vi "setup_lc_db.vi"(4 "shuoming":string, 6 "jsren":string, 7 "zc_luodi_num":string, 8 "didian":string, 9 "yw":string, 11 "id":string) -> (2 "error":errorcluster caption="error out 2")   [LabVIEW 2017, in "Lib_code.lvlib"]
uses:
  Lib_code.lvlib
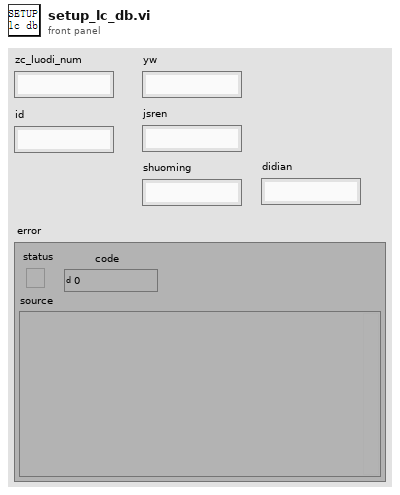
[diagram p1: front panel]
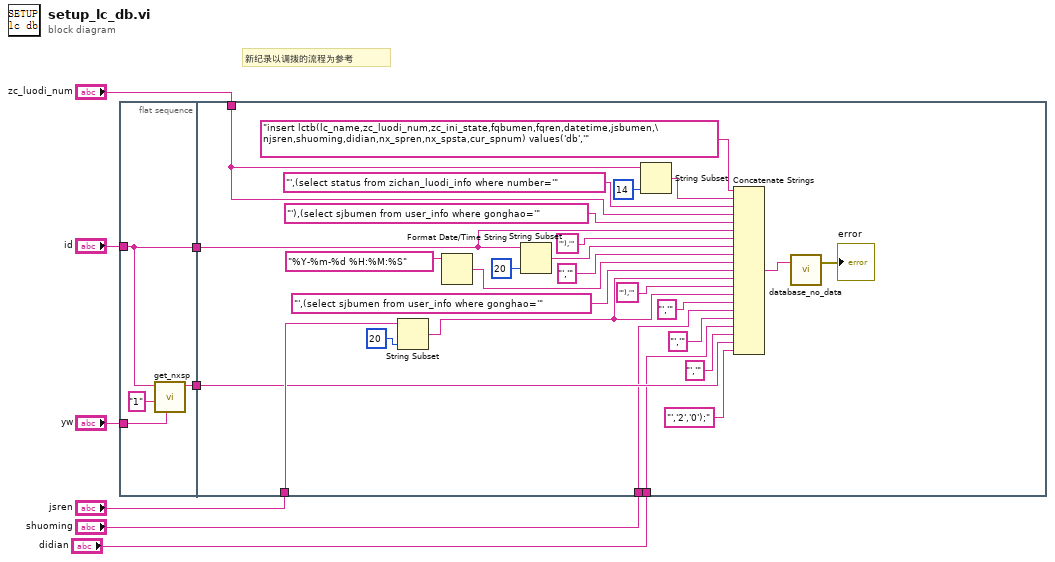
[diagram p0: block diagram]
diagram:
  # "新纪录以调拨的流程为参考"
  n1 = flat-sequence {
    tunnel: "id" -> [w11]
    tunnel: [w11] -> w8
    tunnel: [w12] -> w7
    tunnel: "yw" -> [w10]
    tunnel: w8 -> [w30]
    tunnel: w7 -> [w24]
    tunnel: "zc_luodi_num" -> [w26]
    tunnel: "jsren" -> [w27]
    tunnel: "shuoming" -> [w16]
    tunnel: "didian" -> [w15]
    frame #0 {
      n2 = call "get_nxsp.vi"("yw"=w10, "Cur_state"="1", "fqren"=w11) -> ("sp_gonghao"=w12:string)  [unwired: 6 in, 2 out]
    }
    frame #1 {
      n3 = String Subset(string=w27, length (rest)=20 ("长度（剩余）")) -> (substring=w18:string)  [unwired: 1 in]
      n4 = Format Date/Time String(time format string (%c)="%Y-%m-%d %H:%M:%S" ("时间格式字符串(%c)")) -> (date/time string=w20:string)  [unwired: 2 in]
      n5 = String Subset(string=w30, length (rest)=20 ("长度（剩余）")) -> (substring=w32:string)  [unwired: 1 in]
      n6 = String Subset(string=w26, length (rest)=14 ("长度（剩余）")) -> (substring=w38:string)  [unwired: 1 in]
      n7 = Concatenate Strings("insert lctb(lc_name,zc_luodi_num,zc_ini_state,fqbumen,fqren,datetime,jsbumen,\njsren,shuoming,didian,nx_spren,nx_spsta,cur_spnum) values('db','" ("格式字符串"), w38, "',(select status from zichan_luodi_info where number='" ("字符串"), w26, "'),(select sjbumen from user_info where gonghao='" ("字符串"), w30, "'),'" ("字符串"), w32, "','" ("字符串"), w20, "',(select sjbumen from user_info where gonghao='" ("字符串"), w18, "'),'" ("字符串"), w18, "','" ("字符串"), w16, "','" ("字符串"), w15, "','" ("字符串"), w24, "','2','0');" ("字符串")) -> (w23:string)
      n8 = call "database_no_data.vi"("input"=w23) -> ("error"=→"error":errorcluster)  [unwired: 2 in]
    }
  }
